vi "read 1b prefixed string.vi"(8 "error in (no error)":errorcluster, 11 "TCP Network Connection in":refnum<k5>) -> (0 "error out":errorcluster, 2 "data out":string, 3 "TCP Network Connection out":refnum<k5>)   [LabVIEW 2020]
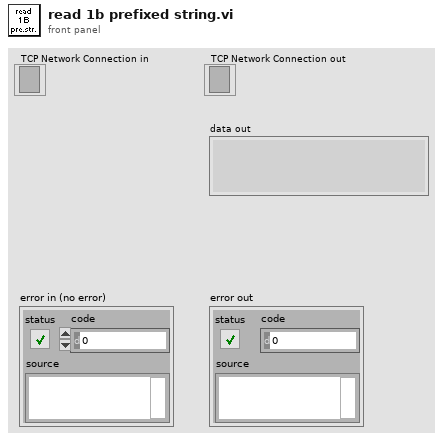
[diagram p1: front panel]
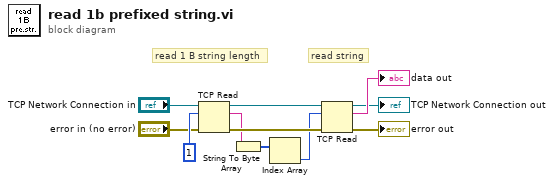
[diagram p0: block diagram]
diagram:
  # "read string"
  # "read 1 B string length"
  n1 = TCP Read(connection ID="TCP Network Connection in", bytes to read=1, error in (no error)="error in (no error)") -> (connection ID out=w7:refnum<k5>, data out=w4:string, error out=w8:errorcluster)  [unwired: 2 in]
  n2 = String To Byte Array(string=w4) -> (unsigned byte array=w5:u8[])
  n3 = Index Array(array=w5) -> (element=w6:u8)  [unwired: 1 in]
  n4 = TCP Read(connection ID=w7, bytes to read=w6, error in (no error)=w8) -> (connection ID out=→"TCP Network Connection out":refnum<k5>, data out=→"data out":string, error out=→"error out":errorcluster)  [unwired: 2 in]
